vi "GEOM_CallGeometry.vi"(0 "Command":string, 11 "error in (no error)":errorcluster) -> (4 "ImmedReplyString":string, 15 "error out":errorcluster)   [LabVIEW 2016]
panel:
  in  "VI path":path=path "/home/ArcVIEW/Modules/GEOM/public/vis"
  in  "AVAPP Cmd Proc":refnum<vi>
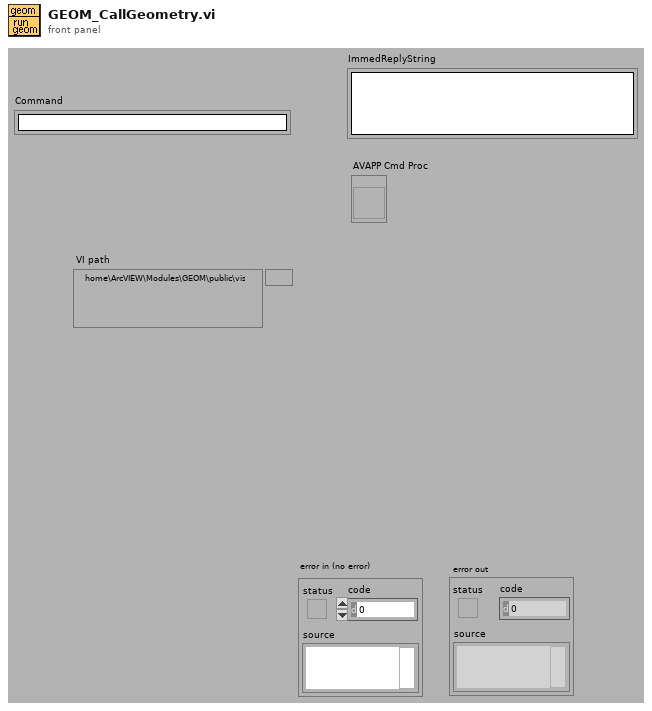
[diagram p1: front panel]
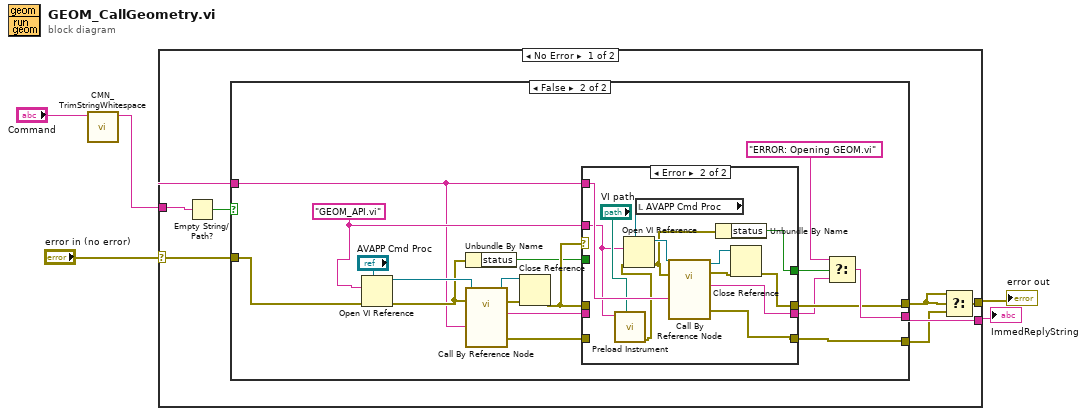
[diagram p0: block diagram]
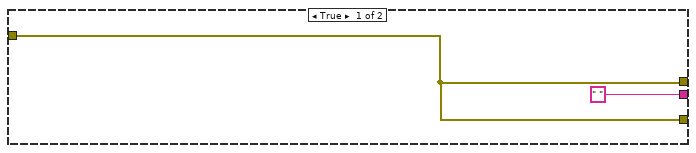
[diagram p2: hidden frame]
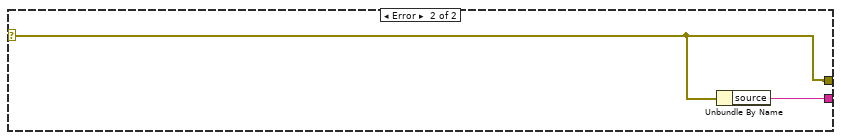
[diagram p4: hidden frame]
diagram:
  n1 = call "CMN_TrimStringWhitespace.vi"("string"="Command") -> ("trimmed string"=w3:string)  [unwired: 1 in, 8 out]
  n2 = case shown="No Error" "error in (no error)" {
    selector: "error in (no error)" -> [w6 w51]
    tunnel: [w12 w50] -> w5
    tunnel: w3 -> [w10 _]
    tunnel: [w7 w51] -> w2
    frame No Error {
      n3 = Empty String/Path?(string/path=w10) -> (empty?=w11:bool)
      n4 = case shown="False" w11 {
        tunnel: [" " w26] -> w12
        tunnel: [w13 w23] -> w9
        tunnel: w6 -> [w13 w30]
        tunnel: w10 -> [_ w15]
        tunnel: [w13 w21] -> w8
        frame True {
        }
        frame False {
          w17 = "GEOM_API.vi"
          n5 = Open VI Reference(type specifier VI Refnum (for type only)="AVAPP Cmd Proc", vi path=w17, error in (no error)=w30) -> (vi reference=w32:refnum<vi>, error out=w27:errorcluster)  [unwired: 3 out]
          n6 = Unbundle By Name(w27) -> ("status"=w20:bool)
          n7 = call-by-ref "Call By Reference Node"(reference=w32, error in=w27, "Cmd"=w15) -> (reference out=w28:refnum<vi>, error out=w29:errorcluster, "ImmedReplyString"=w19:string, 15:"error out"=w22:errorcluster)  [unwired: 13 in]
          n8 = Close Reference(reference=w28, error in (no error)=w29) -> (error out=w24:errorcluster)
          n9 = case shown="Error" w24 {
            tunnel: w24 -> [w36 _]
            tunnel: [w36 w45] -> w23
            tunnel: w22 -> [w35 _]
            tunnel: [w35 w41] -> w21
            tunnel: w20 -> [w33 _]
            tunnel: w19 -> [w34 _]
            tunnel: [w34 w44] -> w18
            tunnel: w17 -> [_ w37]
            tunnel: [w33 w42] -> w16
            tunnel: w15 -> [_ w40]
            frame No Error {
            }
            frame Error {
              n10 = call <vilib>:"Preload Instrument.vi"("VI path"="VI path", "VI name"=w37) -> ("error out"=w38:errorcluster)  [unwired: 1 in, 8 out]
              n11 = local read "AVAPP Cmd Proc"() -> (w49:refnum<vi>)
              n12 = Open VI Reference(type specifier VI Refnum (for type only)=w49, vi path=w37, error in (no error)=w38) -> (vi reference=w48:refnum<vi>, error out=w43:errorcluster)  [unwired: 3 out]
              n13 = call-by-ref "Call By Reference Node"(reference=w48, error in=w43, "Cmd"=w40) -> (reference out=w46:refnum<vi>, error out=w47:errorcluster, "ImmedReplyString"=w44:string, 15:"error out"=w41:errorcluster)  [unwired: 13 in]
              n14 = Unbundle By Name(w43) -> ("status"=w42:bool)
              n15 = Close Reference(reference=w46, error in (no error)=w47) -> (error out=w45:errorcluster)
            }
          }
          n16 = Select(t="ERROR: Opening GEOM.vi", s=w16, f=w18) -> (s? t:f=w26:string)
        }
      }
      n17 = Select(t=w9, s=w9, f=w8) -> (s? t:f=w7:errorcluster)
    }
    frame Error {
      n18 = Unbundle By Name(w51) -> ("source"=w50:string)
    }
  }
  "ImmedReplyString" <- w5
  "error out" <- w2
